vi "Test_SerialNum.vi"() -> ()   [LabVIEW 2017, in "ALMA_10201-10401_O2SensorSim System Explorer.lvlib"]
uses:
  <vilib>/SLSC/Initialize Session without Resources.vi
  <vilib>/SLSC/Close Session.vi
  ALMA_10201-10401_O2SensorSim System Explorer.lvlib
  <vilib>/SLSC/SLSC.lvlib
  <resource>/objmgr/slsc.rc
panel:
  out "Dev.ProductNum":u32
  out "appended array 4":u32[](array[numeric])
  out "appended array 3":string[](array[string])
  out "appended array 2":u32[](array[numeric])
  out "appended array":string[](array[string])
  out "Sys.Modules":refnum<k21>[](array[refnum])
  out "Dev.Modules":refnum<k21>[](array[refnum])
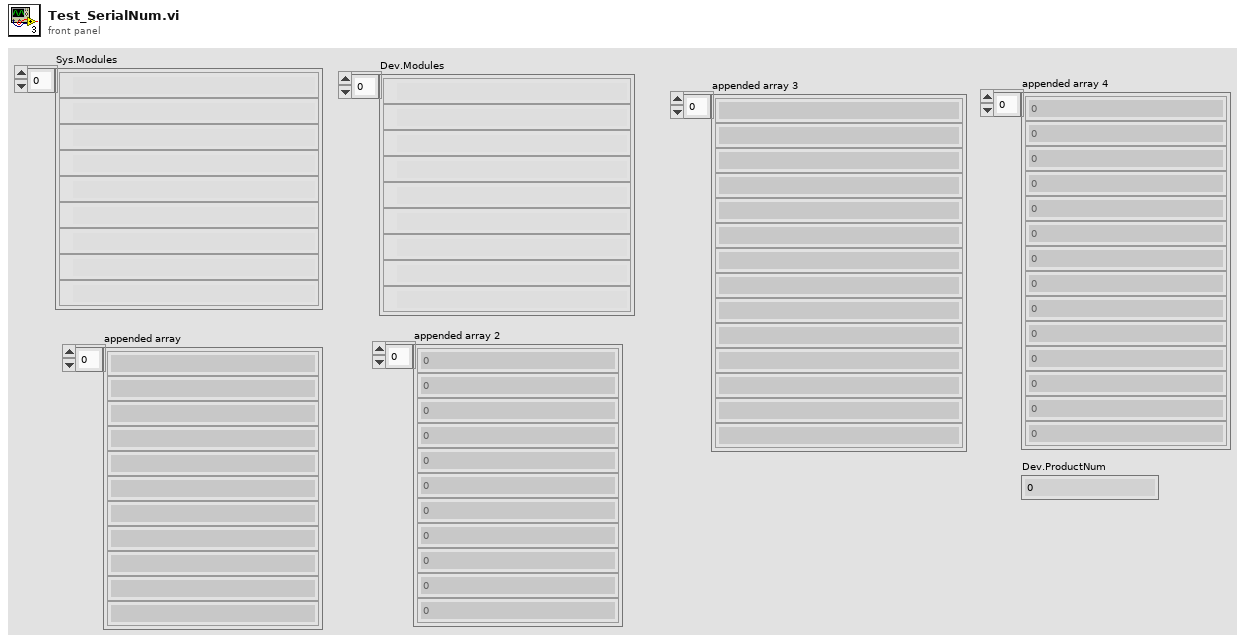
[diagram p1: front panel]
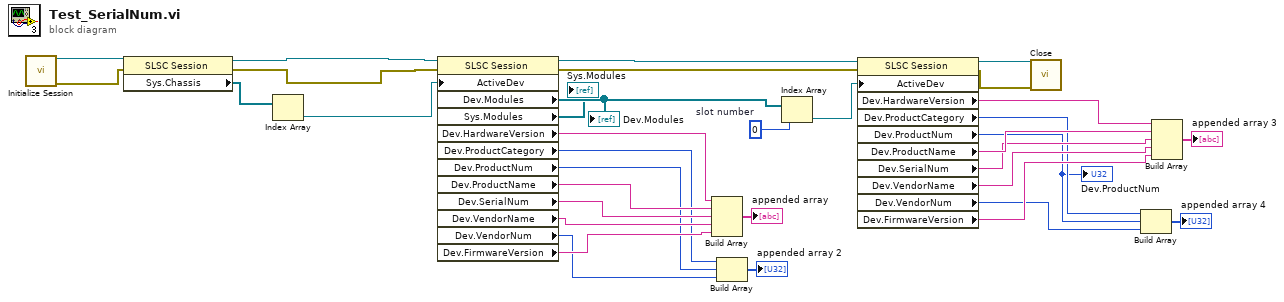
[diagram p0: block diagram]
diagram:
  w20 = 0  # slot number
  n1 = call-poly <vilib>:"Initialize Session.vi"() -> ("session out"=w32:refnum<k21>, "error out"=w31:errorcluster)  [unwired: 14 in]
  n2 = property class="SLSC Session"(reference=w32, error in=w31) -> (reference out=w30:refnum<k21>, error out=w29:errorcluster, "Sys.Chassis"=w33:refnum<k21>[])
  n3 = Index Array(array=w33) -> (element=w27:refnum<k21>)  [unwired: 1 in]
  n4 = property class="SLSC Session"(reference=w30, error in=w29, "ActiveDev"=w27) -> (reference out=w25:refnum<k21>, error out=w24:errorcluster, "Dev.Modules"=w26:refnum<k21>[], "Sys.Modules"=→"Sys.Modules":refnum<k21>[], "Dev.HardwareVersion"=w18:string, "Dev.ProductCategory"=w15:i32, "Dev.ProductNum"=w14:u32, "Dev.ProductName"=w23:string, "Dev.SerialNum"=w22:string, "Dev.VendorName"=w17:string, "Dev.VendorNum"=w13:u32, "Dev.FirmwareVersion"=w16:string)
  "Dev.Modules" <- w26
  n5 = Build Array(w18, w23, w22, w17, w16) -> (→"appended array":string[])
  n6 = Build Array(w15, w14, w13) -> (→"appended array 2":u32[])
  n7 = Index Array(array=w26, index=w20) -> (element=w21:refnum<k21>)
  n8 = property class="SLSC Session"(reference=w25, error in=w24, "ActiveDev"=w21) -> (reference out=w34:refnum<k21>, error out=w28:errorcluster, "Dev.HardwareVersion"=w19:string, "Dev.ProductCategory"=w3:i32, "Dev.ProductNum"=w2:u32, "Dev.ProductName"=w9:string, "Dev.SerialNum"=w8:string, "Dev.VendorName"=w7:string, "Dev.VendorNum"=w1:u32, "Dev.FirmwareVersion"=w6:string)
  "Dev.ProductNum" <- w2
  n9 = call-poly <vilib>:"Close.vi"("session in"=w34, "error in (no error)"=w28) -> ()  [unwired: 13 in, 1 out]
  n10 = Build Array(w3, w2, w1) -> (→"appended array 4":u32[])
  n11 = Build Array(w19, w9, w8, w7, w6) -> (→"appended array 3":string[])
